vi "Ejercicio_15_Escritura_Digital.vi"() -> ()   [LabVIEW 2021]
panel:
  out "XY Graph 2":cluster{dbl[], dbl[]}[](graph)
  in  "stop":bool
  out "Array 2":dbl[](array[numeric])
  out "Array":dbl[](array[numeric])
  out "Waveform Chart":dynamicdata(graph)
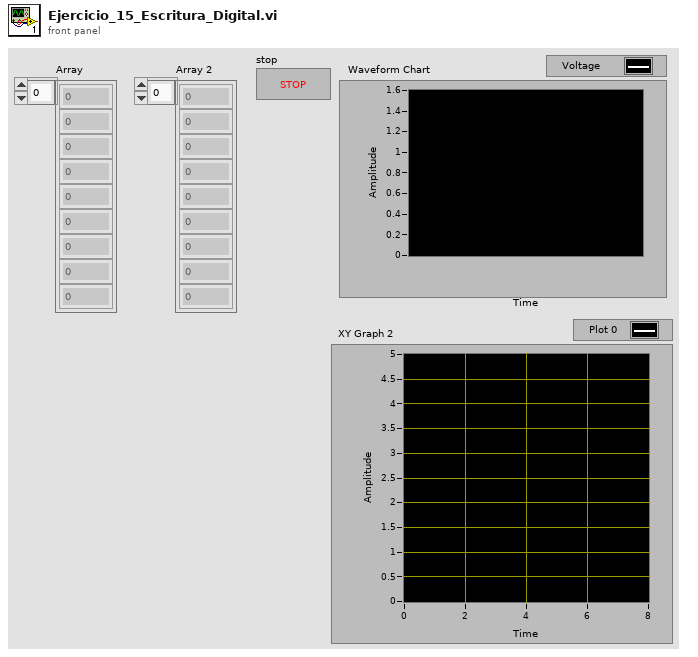
[diagram p1: front panel]
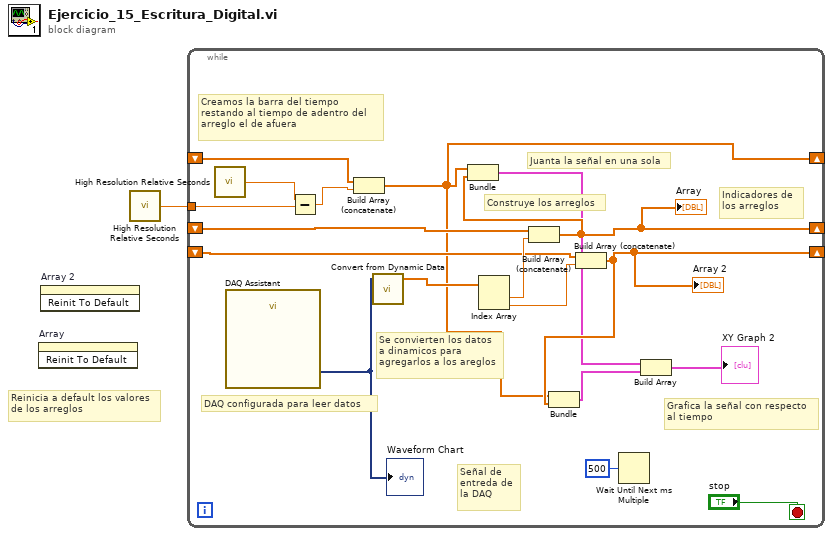
[diagram p0: block diagram]
diagram:
  # "Reinicia a default los valores\nde los arreglos"
  n1 = invoke on="Array" class="Arr (strict)" method="Reinit To Default"() -> ()  [unwired: 3 in, 3 out]
  n2 = invoke on="Array 2" class="Arr (strict)" method="Reinit To Default"() -> ()  [unwired: 3 in, 3 out]
  n3 = call <vilib>:"High Resolution Relative Seconds.vi"() -> ("relative seconds"=w1:dbl)
  n4 = while {
    shift-right: [w8] -> _
    shift-left: _ -> [w16]
    shift-right: [w7] -> _
    shift-left: _ -> [w15]
    tunnel: w1 -> [w10]
    shift-right: [w6] -> _
    shift-left: _ -> [w9]
    stop <- "stop" stop-if-true
    # "Construye los arreglos"
    # "Juanta la señal en una sola"
    # "Indicadores de \nlos arreglos"
    # "Grafica la señal con respecto\nal tiempo"
    # "Señal de \nentreda de \nla DAQ"
    # "Creamos la barra del tiempo\nrestando al tiempo de adentro del \narreglo el de afuera"
    # "Se convierten los datos\na dinamicos para \nagregarlos a los areglos"
    # "DAQ configurada para leer datos"
    n5 = call <vilib>:"High Resolution Relative Seconds.vi"() -> ("relative seconds"=w11:dbl)
    n6 = call "DAQ Assistant"() -> ("data"=w13:dynamicdata)  [unwired: 17 in, 2 out]
    "Waveform Chart" <- w13
    n7 = Subtract(x=w11, y=w10) -> (x-y=w12:dbl)
    n8 = Build Array (concatenate)(w9, w12) -> (w6:dbl[])
    n9 = call "Convert from Dynamic Data"("Dynamic Data Type"=w13) -> ("Array"=w19:dbl[])  [unwired: 3 in]
    n10 = Index Array "Index Array"(array=w19) -> (element #1=w18:dbl, element #2=w17:dbl)  [unwired: 2 in]
    n11 = Build Array (concatenate) "Build Array"(w16, w18) -> (w8:dbl[])
    "Array" <- w8
    n12 = Bundle "Bundle"(w6, w8) -> (w4:cluster{dbl[], dbl[]})  [unwired: 1 in]
    n13 = Build Array (concatenate)(w15, w17) -> (w7:dbl[])
    "Array 2" <- w7
    n14 = Bundle(w6, w7) -> (w5:cluster{dbl[], dbl[]})  [unwired: 1 in]
    n15 = Wait Until Next ms Multiple(millisecond multiple=u32 500) -> ()  [unwired: 1 out]
    n16 = Build Array(w4, w5) -> (→"XY Graph 2":cluster{dbl[], dbl[]}[])
  }
